vi "报警信息.vi"(8 "error in (no error)":errorcluster, 11 "data in":T1) -> (0 "error out":errorcluster)   [LabVIEW 2016, in "超标留样集成.lvlib" / "德润DR803M超标留样.lvlib"]
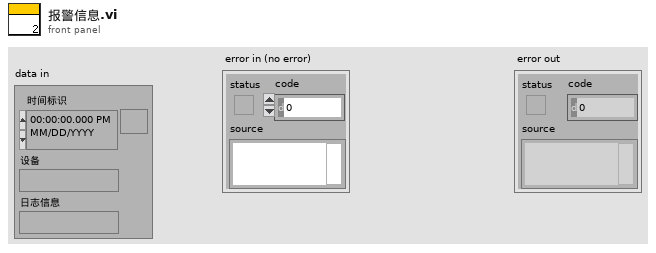
[diagram p1: front panel]
types:
  T1 = cluster{"时间标识":timestamp, "设备":string, "日志信息":string}
  T2 = typedef "报警信息字段定义.ctl" = cluster{"时间":timestamp, "参数":string, "报警信息":string, "备注":string}
  T3 = typedef "数据库类型.ctl" = enum16{"Access", "SQLite"}
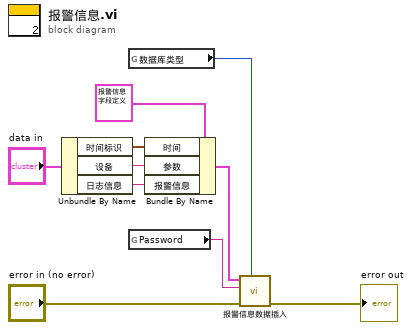
[diagram p0: block diagram]
diagram:
  n1 = Unbundle By Name("data in") -> ("时间标识"=w8:timestamp, "设备"=w7:string, "日志信息"=w6:string)
  n2 = global read "断电保存全局.vi" "数据库类型"() -> (w4:T3)
  n3 = global read "断电保存全局.vi" "Password"() -> (w1:string)
  n4 = Bundle By Name(cluster=T2 {"时间"=timestamp(0 s since 1904-01-01), "参数"="水样测试", "报警信息"="N", "备注"=""} ("data"), "时间"=w8, "参数"=w7, "报警信息"=w6) -> (w5:T2)
  n5 = call "报警信息数据插入.vi"("data"=w5, "Password"=w1, "错误输入（无错误）"="error in (no error)", "数据库类型"=w4) -> ("错误输出"=→"error out":errorcluster)  [unwired: 6 in]
